vi "Show Current Location Write.vi"(4 "error in (no error)":errorcluster, 5 "Value":bool, 6 "Container State":T2, 7 "Display State In":T1) -> (0 "error out":errorcluster, 3 "Display State Out":T1)   [LabVIEW 2018, in "Waveform Control.xctl"]
uses:
  Waveform Control.xctl
  <vilib>/_xctls/Container State.ctl
  Controls/State.ctl
  Controls/Volatile State Ops.ctl
  <vilib>/_xctls/XControlSupport.lvlib
panel:
  # "Replace the Value Control below with a Control of desired type.\nDo not remove this Control or the others from the connector pane.\nDo not change the connector pane pattern.\nThe Value control should always be the third terminal from top on the input side in the connector pane."
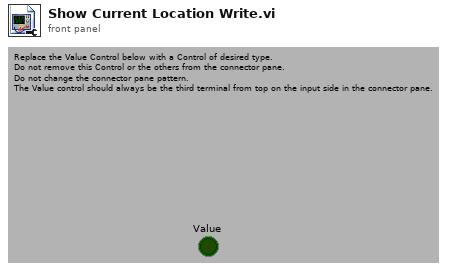
[diagram p1: front panel]
types:
  T1 = typedef "Waveform Control.xctl/State.ctl" = cluster{"Name":string}
  T2 = typedef "XControlSupport.lvlib/Container State.ctl" = cluster{"Indicator?":bool, "Run Mode?":bool, " Refnum":refnum<vi>}
  T3 = typedef "Waveform Control.xctl/Volatile State Ops.ctl" = enum16{"Read", "Write", "Update State from Data"}
  T4 = typedef "Waveform Control.xctl/Waveform State.ctl" = cluster{"Show Axes":bool, "Show Y=0":bool, "Controls":T5, "Show Current Location":bool, "Current Location":i32, "dt":dbl, "t0":timestamp, "Amplitude Format String":string}
  T5 = typedef "Waveform Control.xctl/FP Controls.ctl" = cluster{"Type":T6, "Periods":dbl, "Points":i32, "Offset":dbl, "Amplitdue":dbl, "Starting Phase":dbl, "func":string}
  T6 = typedef "Waveform Control.xctl/Function Types.ctl" = enum16{"Level", "Sine", "Triangle", "Ramp", "Saw Tooth", "Square", "Function"}
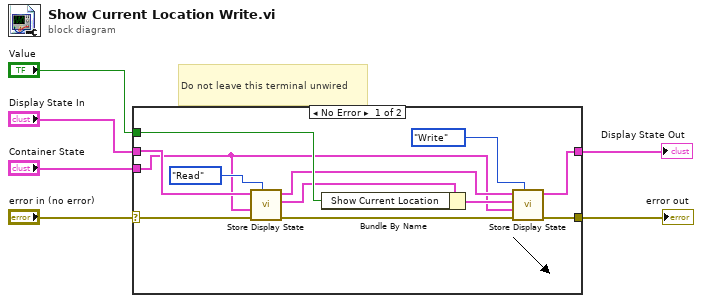
[diagram p0: block diagram]
diagram:
  # "Do not leave this terminal unwired"
  n1 = case shown="No Error" "error in (no error)" {
    selector: "error in (no error)" -> [w17 w19]
    tunnel: [w10 w19] -> w5
    tunnel: "Display State In" -> [w16 w20]
    tunnel: [w9 w20] -> w3
    tunnel: "Value" -> [w18 _]
    tunnel: "Container State" -> [w7 _]
    frame No Error {
      n2 = call "Store Display State.vi"("Operation In"=Volatile_State_Ops."Read" ("Operation"), "Error In (no Error) In"=w17, "Container State In"=w7, "State In"=w16) -> ("Error Out"=w11:errorcluster, "Waveform State Out"=w15:T4, "Display State Out"=w12:T1)  [unwired: 2 in, 3 out]
      n3 = Bundle By Name(cluster=w15, "Show Current Location"=w18) -> (w13:T4)
      n4 = call "Store Display State.vi"("Operation In"=Volatile_State_Ops."Write" ("Operation"), "Error In (no Error) In"=w11, "Container State In"=w7, "Waveform State In"=w13, "State In"=w12) -> ("Error Out"=w10:errorcluster, "Display State Out"=w9:T1)  [unwired: 1 in, 4 out]
    }
    frame Error {
    }
  }
  "error out" <- w5
  "Display State Out" <- w3
